vi "is_valid.vi"(11 "Client in":refnum<class "Client.lvclass">) -> (2 "valid-ref?":bool)   [LabVIEW 2020, in "reqwest.lvlib" / "Client.lvclass"]
uses:
  Client.lvclass
  Client.lvclass/Client.ctl
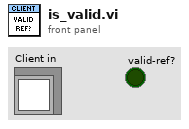
[diagram p1: front panel]
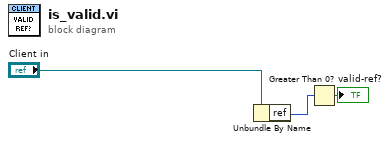
[diagram p0: block diagram]
diagram:
  n1 = Unbundle By Name("Client in") -> ("ref"=w2:u64)
  n2 = Greater Than 0?(x=w2) -> (x > 0?=→"valid-ref?":bool)
